vi "Load Cell Sensitivity DAO.vi"(7 "Config Ref  In":T2, 8 "error in (no error)":errorcluster, 9 "Load Cell Sensitivity Offset In":T1, 10 "LBCB Number":T3, 11 "Actions":T4) -> (0 "error out":errorcluster, 1 "Load Cell Sensitivity Offsets Out":T1, 6 "Config Ref Out":T2)   [LabVIEW 2009]
uses:
  Metadata/Persistant DAO Actions.ctl
  Metadata/LBCB Number.ctl
  Metadata/Actuator Point.ctl
  <vilib>/Utility/config.llb/Config Data RefNum.ctl
  <vilib>/Utility/config.llb/NI_LVConfig.lvlib
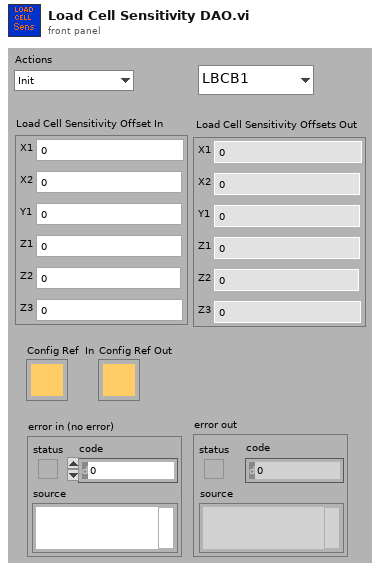
[diagram p1: front panel]
types:
  T1 = typedef "Actuator Point.ctl" = cluster{"X1":dbl, "X2":dbl, "Y1":dbl, "Z1":dbl, "Z2":dbl, "Z3":dbl}
  T2 = typedef "NI_LVConfig.lvlib/Config Data RefNum.ctl" = refnum<k1>
  T3 = typedef "LBCB Number.ctl" = enum16{"LBCB1", "LBCB2"}
  T4 = typedef "Persistant DAO Actions.ctl" = enum16{"Init", "Get", "Set", "Load", "Save"}
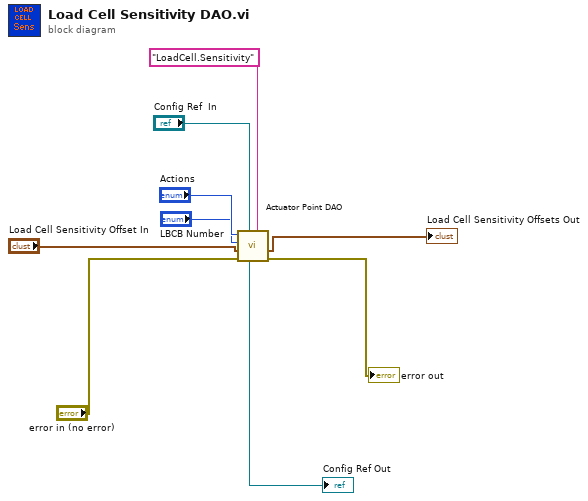
[diagram p0: block diagram]
diagram:
  n1 = call "Actuator Point DAO.vi"("section"="LoadCell.Sensitivity", "Config Ref  In"="Config Ref  In", "error in (no error)"="error in (no error)", "Point In"="Load Cell Sensitivity Offset In", "LBCB Number"="LBCB Number", "Actions"="Actions") -> ("error out"=→"error out":errorcluster, "Point Out"=→"Load Cell Sensitivity Offsets Out":T1, "Config Ref Out"=→"Config Ref Out":T2)  [unwired: 3 out]
